vi "Encoder Distance.vi"() -> ()   [LabVIEW 2016]
panel:
  out "W)(331 3nc0d3r":dbl
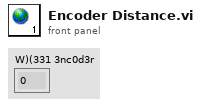
[diagram p1: front panel]
diagram:
